vi "Dashboard.vi"() -> ()   [LabVIEW 2024, in "UIs Handler.lvlib"]
uses:
  UIs Handler.lvlib
  Custom Controls/Select Signal from UI.ctl
  Custom Controls/Reset Button.ctl
  Custom Controls/Save Button.ctl
  Custom Controls/Start Button.ctl
  States.ctl
panel:
  out "Temp Ind":dbl=120.0 format="%-#2.1f"
  out "S":i32=99
  out "M":dbl=99.0
  out "H":dbl=99.0
  in  "Start Counter":T1
  in  "Save Counter":T2
  in  "Reset Counter":T3
  out "Waveform Chart - Light":T4(graph)
  in  "Select Signal":T5 {"Value 8" format="%#.2g"; "Value 7" format="%#.2g"; "Value 6" format="%#.2g"; "Value 5" format="%#.2g"; "Value 4" format="%#.2g"; "Value 3" format="%#.2g"; "Value 2" format="%#.2g"; "Value 1" format="%.2g"}
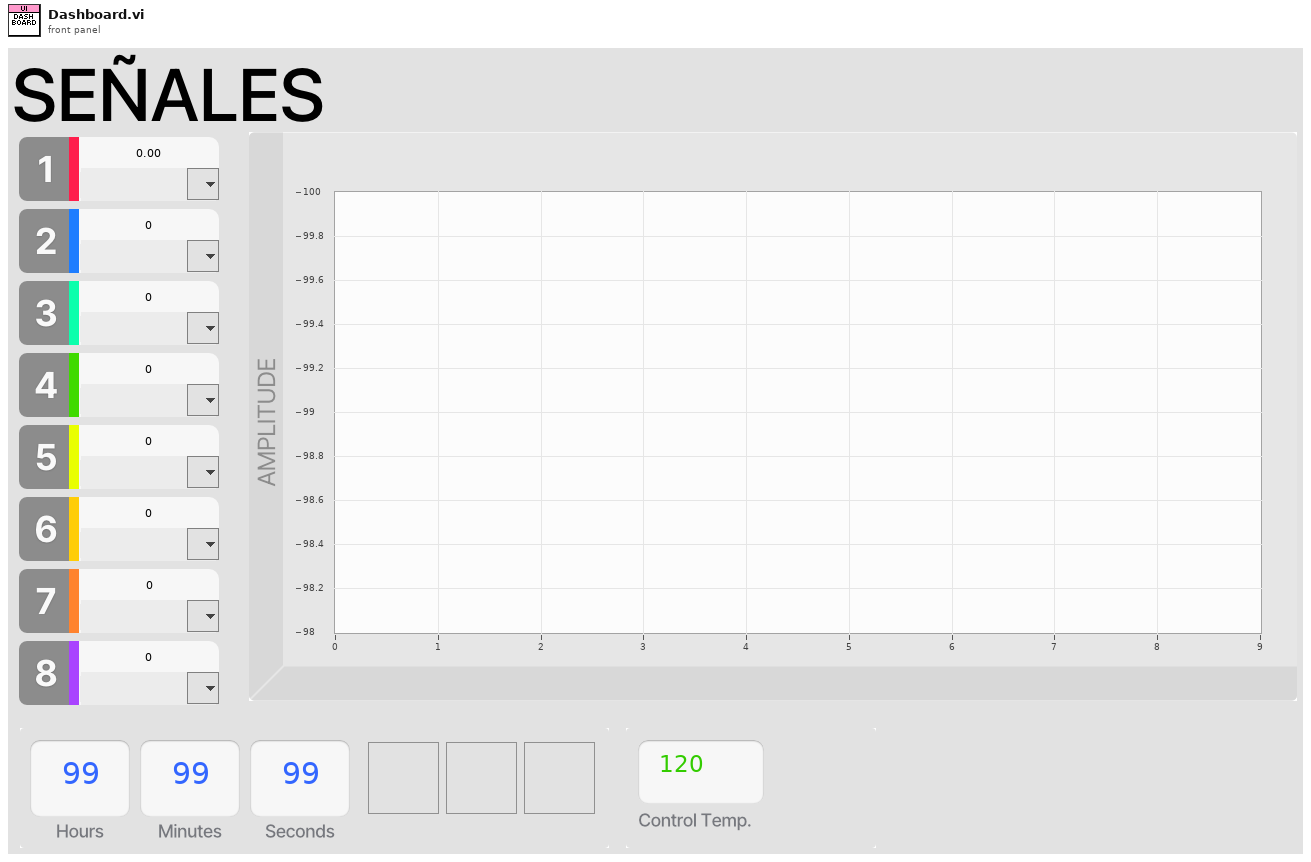
[diagram p1: front panel]
types:
  T1 = typedef "UIs Handler.lvlib/Start Button.ctl" = bool
  T2 = typedef "UIs Handler.lvlib/Save Button.ctl" = bool
  T3 = typedef "UIs Handler.lvlib/Reset Button.ctl" = bool
  T4 = cluster{"Signals[0]":dbl, "Signals[1]":dbl, "Signals[2]":dbl, "Signals[3]":dbl, "Signals[4]":dbl, "Signals[5]":dbl, "Signals[6]":dbl, "Signals[7]":dbl, "Signals[8]":dbl, "Signals[9]":dbl, "Signals[10]":dbl, "Signals[11]":dbl, "Signals[12]":dbl, "Signals[13]":dbl, "Signals[14]":dbl, "Signals[15]":dbl, "Signals[16]":dbl, "Signals[17]":dbl, "Signals[18]":dbl, "Signals[19]":dbl}
  T5 = typedef "UIs Handler.lvlib/Select Signal from UI.ctl" = cluster{"Signal 1":string, "Value 1":dbl, "Value 2":dbl, "Signal 2":string, "Value 3":dbl, "Signal 3":string, "Value 4":dbl, "Signal 4":string, "Value 5":dbl, "Signal 5":string, "Value 6":dbl, "Signal 6":string, "Value 7":dbl, "Signal 7":string, "Value 8":dbl, "Signal 8":string}
  T6 = typedef "UIs Handler.lvlib/States.ctl" = enum16{"Init", "Wait for Event", "Error", "Read Image", "Close"}
  T7 = typedef "UIs Handler.lvlib/Broadcast Events--cluster.ctl" = cluster{"Module Did Init":refnum<user-event>, "Status Updated":refnum<user-event>, "Error Reported":refnum<user-event>, "Module Did Stop":refnum<user-event>, "Update Module Execution Status":refnum<user-event>, "Update Data":refnum<user-event>}
  T8 = cluster{"Signals[0]":dbl, "Signals[1]":dbl, "Signals[2]":dbl, "Signals[3]":dbl, "Signals[4]":dbl, "Signals[5]":dbl, "Signals[6]":dbl, "Signals[7]":dbl, "Signals[8]":dbl, "Signals[9]":dbl, "Signals[10]":dbl, "Signals[11]":dbl, "Signals[12]":dbl, "Signals[13]":dbl, "Signals[14]":dbl, "Signals[15]":dbl, "Signals[16]":dbl, "Signals[17]":dbl, "Signals[18]":dbl, "Signals[19]":dbl}[]
  T9 = cluster{"[0]":dbl, "[1]":dbl, "[2]":dbl, "[3]":dbl, "[4]":dbl, "[5]":dbl, "[6]":dbl, "[7]":dbl, "[8]":dbl, "[9]":dbl, "[10]":dbl, "[11]":dbl, "[12]":dbl, "[13]":dbl, "[14]":dbl, "[15]":dbl, "[16]":dbl, "[17]":dbl, "[18]":dbl, "[19]":dbl}
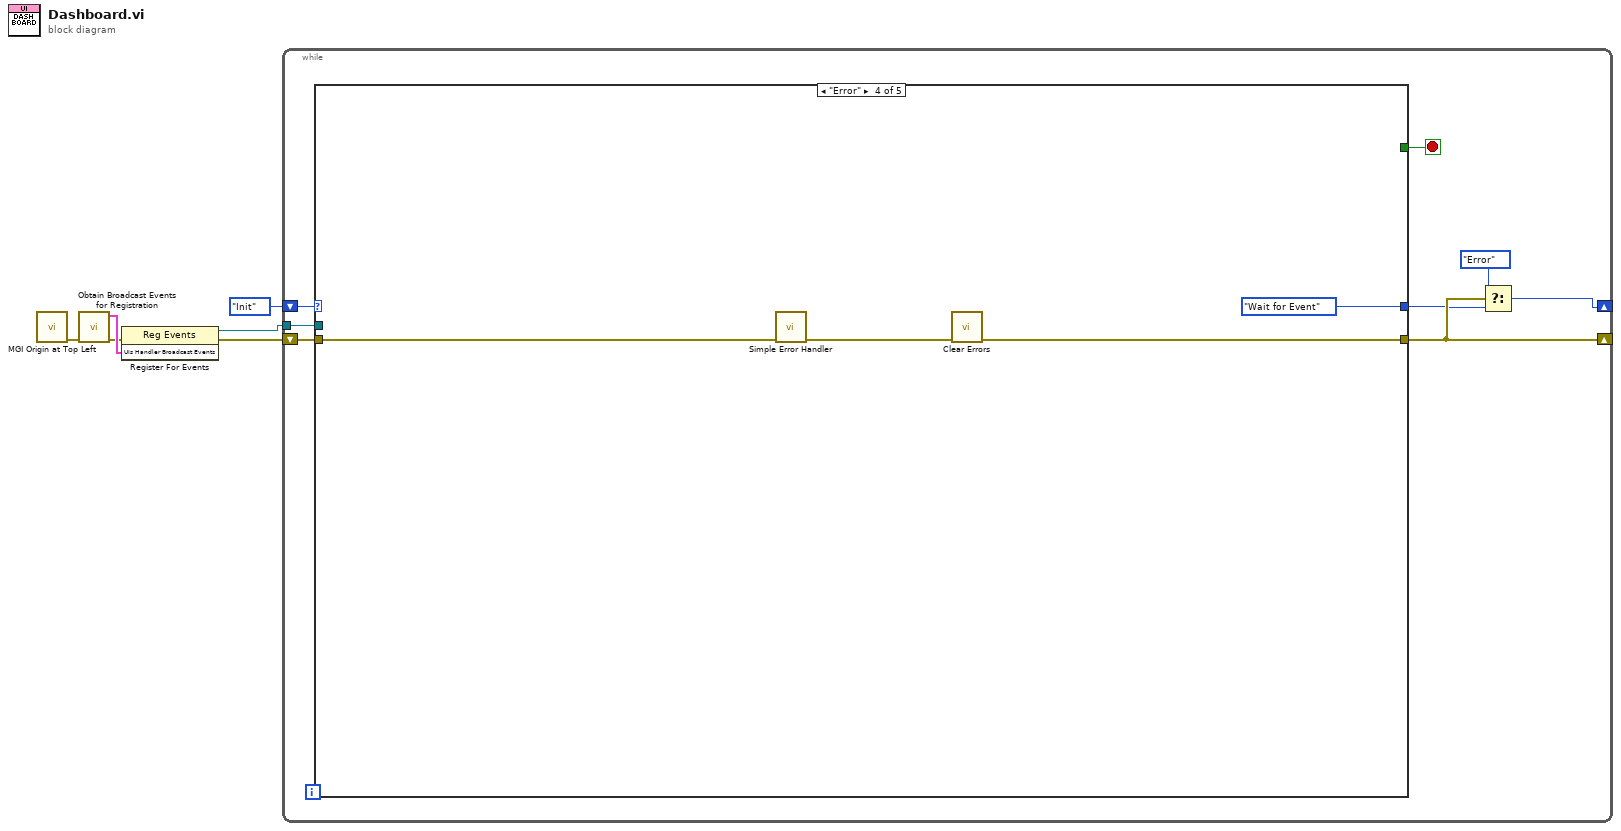
[diagram p0: block diagram]
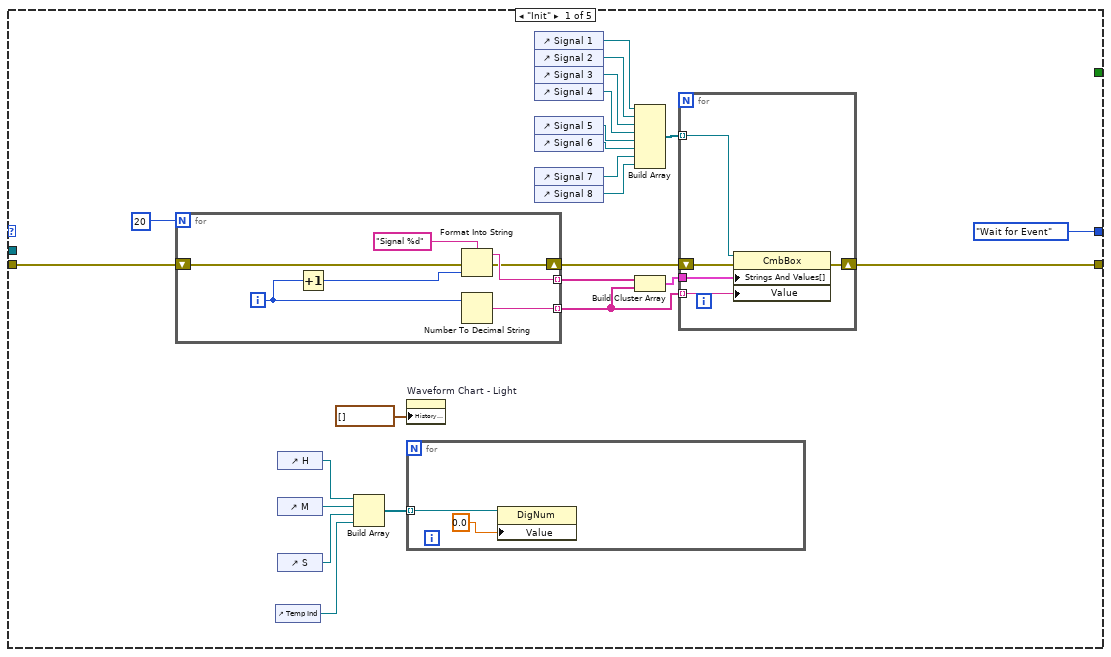
[diagram p2: hidden frame]
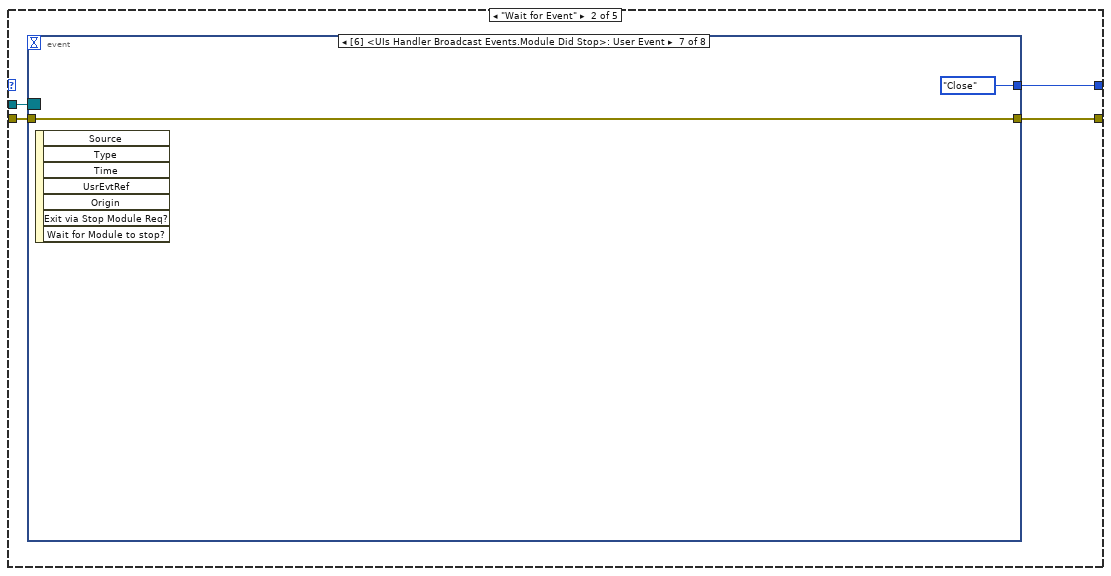
[diagram p3: hidden frame]
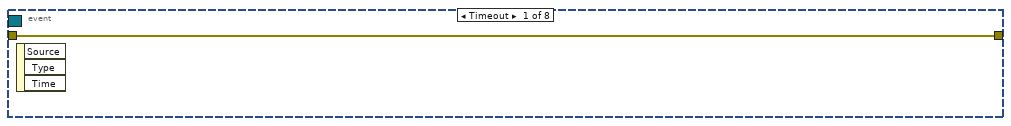
[diagram p4: hidden frame]
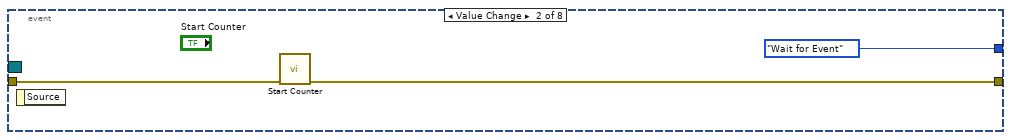
[diagram p5: hidden frame]
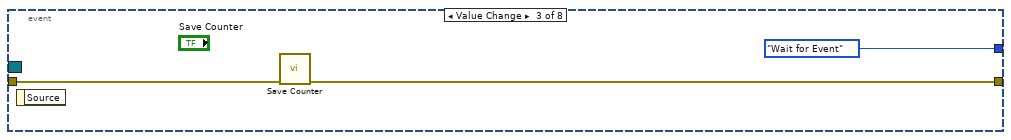
[diagram p6: hidden frame]
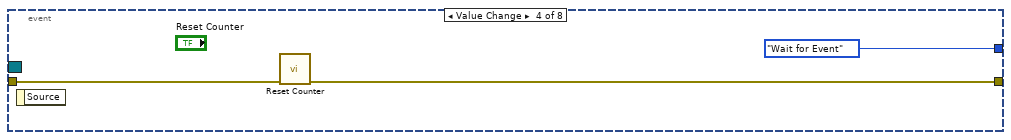
[diagram p7: hidden frame]
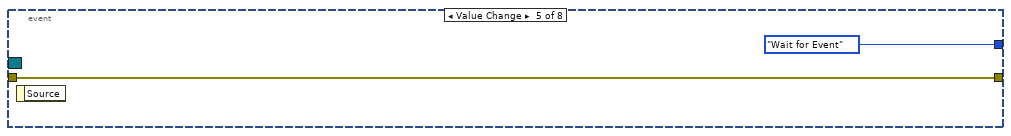
[diagram p8: hidden frame]
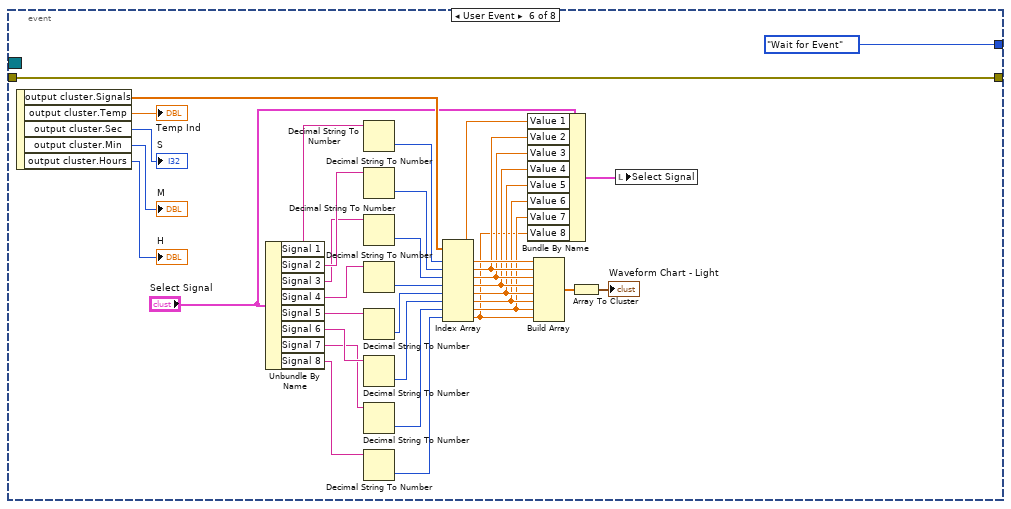
[diagram p9: hidden frame]
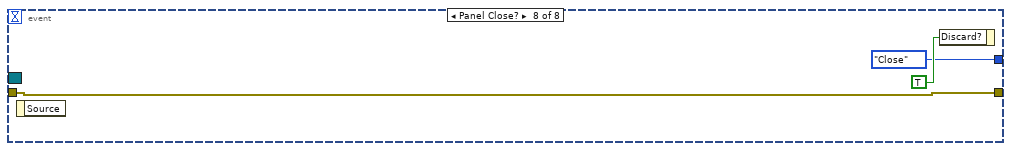
[diagram p10: hidden frame]
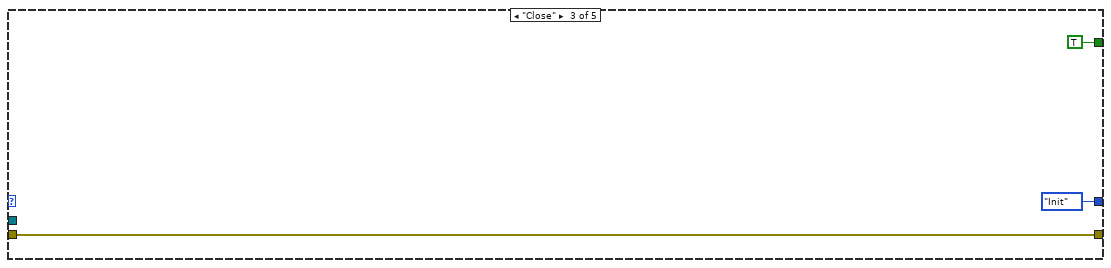
[diagram p11: hidden frame]
diagram:
  n1 = call <userlib>:"MGI Origin at Top Left.vi"() -> ("Error Out"=w5:errorcluster)  [unwired: 9 in, 1 out]
  n2 = call "Obtain Broadcast Events for Registration.vi"("error in"=w5) -> ("error out"=w2:errorcluster, "UIs Handler Broadcast Events"=w4:T7)  [unwired: 8 in, 1 out]
  n3 = register-events(error in=w2, w4) -> (reference out=w3:refnum<event-registration>, error out=w1:errorcluster)  [unwired: 1 in]
  n4 = while {
    shift-right: [w8] -> _
    shift-left: States."Init" ("States") -> [w14]
    shift-right: [w10] -> _
    shift-left: w1 -> [w12]
    tunnel: w3 -> [w11]
    stop <- w13 stop-if-true
    n5 = case shown="\"Error\"" w14 {
      selector: w14 -> [_ _ _ _ w116]
      tunnel: [States."Wait for Event" ("States") w55 States."Init" ("States") States."Wait for Event" ("States") w116] -> w9
      tunnel: [_ _ TRUE _ _] -> w13
      tunnel: w12 -> [w27 w53 w108 w113 w115]
      tunnel: [w25 w52 w108 w111 w115] -> w10
      tunnel: w11 -> [_ w54 _ _ _]
      frame "Init" {
        n6 = for {
          N: 20 -> [_]
          tunnel: [w49] -> w22 mode=indexing
          shift-right: [w47] -> w26
          shift-left: w27 -> [w48]
          tunnel: [w45] -> w15 mode=indexing
          i -> [w46]
          n7 = Increment(x=w46) -> (x+1=w51:i32)
          n8 = Format Into String(format string="Signal %d", error in=w48, w51) -> (resulting string=w49:string, error out=w47:errorcluster)  [unwired: 1 in]
          n9 = Number To Decimal String(number=w46) -> (decimal integer string=w45:string)  [unwired: 1 in]
        }
        n10 = control-ref of="Temp Ind"() -> (w18:refnum<vi>)
        n11 = control-ref of="H"() -> (w21:refnum<vi>)
        n12 = control-ref of="M"() -> (w20:refnum<vi>)
        n13 = control-ref of="S"() -> (w19:refnum<vi>)
        n14 = Build Array(w21, w20, w19, w18) -> (w17:refnum<vi>[])
        n15 = property on="Waveform Chart - Light" class="WFChart (strict)"("History Data"=T8 []) -> ()  [unwired: 2 in, 2 out]
        n16 = for {
          tunnel: w17 -> [w39] mode=indexing
          n17 = property class="DigNum"(reference=w39, "Value"=0.0) -> ()  [unwired: 1 in, 2 out]
        }
        n18 = control-ref of="Signal 1"() -> (w37:refnum<vi>)
        n19 = control-ref of="Signal 2"() -> (w36:refnum<vi>)
        n20 = control-ref of="Signal 3"() -> (w35:refnum<vi>)
        n21 = control-ref of="Signal 4"() -> (w34:refnum<vi>)
        n22 = control-ref of="Signal 5"() -> (w33:refnum<vi>)
        n23 = control-ref of="Signal 6"() -> (w32:refnum<vi>)
        n24 = control-ref of="Signal 7"() -> (w31:refnum<vi>)
        n25 = control-ref of="Signal 8"() -> (w30:refnum<vi>)
        n26 = Build Array(w37, w36, w35, w34, w33, w32, w31, w30) -> (w24:refnum<vi>[])
        n27 = Build Cluster Array(w22, w15) -> (w29:cluster{string, string}[])
        n28 = for {
          tunnel: w24 -> [w44] mode=indexing
          tunnel: w29 -> [w43]
          shift-right: [w41] -> w25
          shift-left: w26 -> [w42]
          tunnel: w15 -> [w40] mode=indexing
          n29 = property class="CmbBox"(reference=w44, error in=w42, "Strings And Values[]"=w43, "Value"=w40) -> (error out=w41:errorcluster)  [unwired: 1 out]
        }
      }
      frame "Wait for Event" {
        n30 = event shown="[6] <UIs Handler Broadcast Events.Module Did Stop>: User Event" {
          selector: w54 -> [_ _ _ _ _ _ _ _]
          dyn-events: _ -> [_ _ _ _ _ _ _ _]
          timeout: _ -> [_ _ _ _ _ _ _ _]
          tunnel: [_ States."Wait for Event" ("States") States."Wait for Event" ("States") States."Wait for Event" ("States") States."Wait for Event" ("States") States."Wait for Event" ("States") States."Close" ("States") States."Close" ("States")] -> w55
          tunnel: w53 -> [w56 w58 w61 w64 w66 w96 w104 w105]
          tunnel: [w56 w57 w60 w63 w66 w96 w104 w105] -> w52
          event Timeout {
            n31 = event-data() -> ()  [unwired: 1 in, 3 out]
          }
          event Value Change {
            n32 = event-data() -> ()  [unwired: 1 in, 1 out]
            n33 = call "Start Counter.vi"("error in"=w58) -> ("error out"=w57:errorcluster)  [unwired: 10 in]
          }
          event Value Change {
            n34 = event-data() -> ()  [unwired: 1 in, 1 out]
            n35 = call "Save Counter.vi"("error in"=w61) -> ("error out"=w60:errorcluster)  [unwired: 10 in]
          }
          event Value Change {
            n36 = event-data() -> ()  [unwired: 1 in, 1 out]
            n37 = call "Reset Counter.vi"("error in"=w64) -> ("error out"=w63:errorcluster)  [unwired: 10 in]
          }
          event Value Change {
            n38 = event-data() -> ()  [unwired: 1 in, 1 out]
          }
          event User Event {
            n39 = event-data() -> ("output cluster.Signals"=w95:dbl[], "output cluster.Temp"=→"Temp Ind":dbl, "output cluster.Sec"=→"S":i32, "output cluster.Min"=→"M":i32, "output cluster.Hours"=→"H":i32)  [unwired: 1 in]
            n40 = Unbundle By Name("Select Signal") -> ("Signal 1"=w94:string, "Signal 2"=w91:string, "Signal 3"=w89:string, "Signal 4"=w88:string, "Signal 5"=w87:string, "Signal 6"=w86:string, "Signal 7"=w85:string, "Signal 8"=w84:string)
            n41 = Decimal String To Number(string=w94) -> (number=w93:i32)  [unwired: 2 in, 1 out]
            n42 = Decimal String To Number(string=w91) -> (number=w90:i32)  [unwired: 2 in, 1 out]
            n43 = Decimal String To Number(string=w89) -> (number=w83:i32)  [unwired: 2 in, 1 out]
            n44 = Decimal String To Number(string=w88) -> (number=w82:i32)  [unwired: 2 in, 1 out]
            n45 = Decimal String To Number(string=w87) -> (number=w81:i32)  [unwired: 2 in, 1 out]
            n46 = Decimal String To Number(string=w86) -> (number=w80:i32)  [unwired: 2 in, 1 out]
            n47 = Decimal String To Number(string=w85) -> (number=w79:i32)  [unwired: 2 in, 1 out]
            n48 = Decimal String To Number(string=w84) -> (number=w78:i32)  [unwired: 2 in, 1 out]
            n49 = Index Array(array=w95, index #1=w93, index #2=w90, index #3=w83, index #4=w82, index #5=w81, index #6=w80, index #7=w79, index #8=w78) -> (element #1=w76:dbl, element #2=w75:dbl, element #3=w74:dbl, element #4=w73:dbl, element #5=w72:dbl, element #6=w71:dbl, element #7=w70:dbl, element #8=w69:dbl)
            n50 = Bundle By Name(cluster="Select Signal", "Value 1"=w76, "Value 2"=w75, "Value 3"=w74, "Value 4"=w73, "Value 5"=w72, "Value 6"=w71, "Value 7"=w70, "Value 8"=w69) -> (w68:T5)
            n51 = Build Array(w76, w75, w74, w73, w72, w71, w70, w69) -> (w92:dbl[])
            n52 = Array To Cluster(array=w92) -> (cluster=→"Waveform Chart - Light":T9)
            n53 = local write "Select Signal"(w68) -> ()
          }
          event User Event {
            n54 = event-data() -> ()  [unwired: 1 in, 7 out]
          }
          event Panel Close? {
            n55 = event-data() -> ()  [unwired: 1 in, 1 out]
            n56 = event-data("Discard?"=TRUE) -> ()  [unwired: 1 in, 1 out]
          }
        }
      }
      frame "Close" {
      }
      frame "Error" {
        n57 = call <vilib>:"Simple Error Handler.vi"("error in (no error)"=w113) -> ("error out"=w112:errorcluster)  [unwired: 4 in, 4 out]
        n58 = call <vilib>:"Clear Errors.vi"("error in (no error)"=w112) -> ("error out"=w111:errorcluster)  [unwired: 5 in, 1 out]
      }
      frame Default {
      }
    }
    n59 = Select(t=States."Error", s=w10, f=w9) -> (s? t:f=w8:T6)
  }
